vi "Simple.vi"(8 "Error In":errorcluster, 10 "Username":string, 11 "Password":string) -> (0 "Error Out":errorcluster)   [LabVIEW 2013, in "LVH-Nest.lvlib"]
uses:
  LVH-Nest.lvlib
  Private/Type Defs/Thermostat Mode.ctl
panel:
  in  "Thermostat Mode":T1
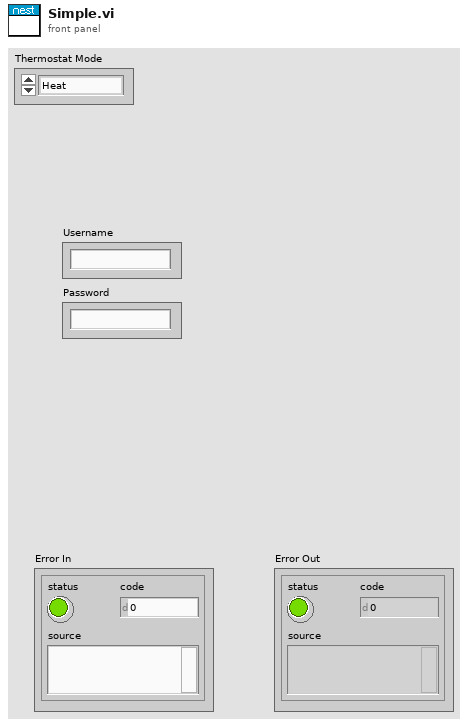
[diagram p1: front panel]
types:
  T1 = typedef "LVH-Nest.lvlib/Thermostat Mode.ctl" = enum16{"Heat", "Cool", "Heat / Cool"}
  T2 = typedef "LVH-Nest.lvlib/Nest Config.ctl" = cluster{"Client Handle":T3, "Session Data":T4}
  T3 = typedef "LabVIEWHTTPClient.lvlib/ClientHandle.ctl" = refnum<k1>
  T4 = typedef "LVH-Nest.lvlib/Session Data.ctl" = cluster{"is_superuser":bool, "is_staff":bool, "urls":cluster{"transport_url":string, "rubyapi_url":string, "weather_url":string, "log_upload_url":string, "support_url":string}, "limits":cluster{"thermostats_per_structure":u32, "structures":u32, "thermostats":u32, "smoke_detectors":u32, "smoke_detectors_per_structure":u32}, "access_token":string, "userid":string, "expires_in":string, "email":string, "user":string, "language":string}
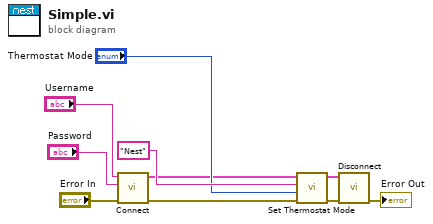
[diagram p0: block diagram]
diagram:
  n1 = call "Connect.vi"("Error In"="Error In", "Password"="Password", "Username"="Username") -> ("Error Out"=w1:errorcluster, "Nest Config"=w2:T2)  [unwired: 7 in]
  n2 = call "Set Thermostat Mode.vi"("Error In"=w1, "Thermostat Mode"="Thermostat Mode", "Device Name"="Nest", "Nest Config"=w2) -> ("Error Out"=w5:errorcluster, "Nest Config"=w6:T2)  [unwired: 6 in]
  n3 = call "Disconnect.vi"("Error In"=w5, "Nest Config"=w6) -> ("Error Out"=→"Error Out":errorcluster)  [unwired: 9 in]
